vi "Periodic Tasks.vi"(8 "error in":errorcluster) -> ()   [LabVIEW 2013]
doc: "This VI runs in parallel to other tasks. It can contain as many user-defined periodic loops as you need. These can carry out PID or other sorts of timed response."
uses:
  Control 5.ctl
  <vilib>/Rock Robotics/SystemInterfaces/Utilities/FPGA_UtilitiesLED Source.ctl
  <vilib>/Rock Robotics/SystemInterfaces/Utilities/FPGA_UtilitiesLED State.ctl
  Robot Global Data.vi
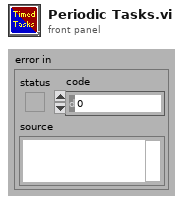
[diagram p1: front panel]
types:
  T1 = typedef "Control 5.ctl" = enum16{"Init", "SetValue", "Disable"}
  T2 = typedef "FPGA_UtilitiesLED State.ctl" = enum16{"Off", "On", "Toggle"}
  T3 = typedef "FPGA_UtilitiesLED Source.ctl" = enum16{"User LED", "FPGA LED"}
  T4 = typedef "WPI_CompressorDevRef.ctl" = cluster{"DevStatus":errorcluster, "DigitalInputDevRef":T5, "RelayDevRef":T8}
  T5 = typedef "WPI_DigitalInputDevRef.ctl" = cluster{"DevStatus":errorcluster, "DIO Channel":T6, "Digital Module":T7}
  T6 = typedef "FPGA_DIOChannel.ctl" = enum8{"DIO 1", "DIO 2", "DIO 3", "DIO 4", "DIO 5", "DIO 6", "DIO 7", "DIO 8", "DIO 9", "DIO 10", "DIO 11", "DIO 12", "DIO 13", "DIO 14", "Invalid"}
  T7 = typedef "FPGA_TypedefDigitalModule.ctl" = enum16{"Digital Module 1", "Digital Module 2"}
  T8 = typedef "WPI_RelayDevRef.ctl" = cluster{"DevStatus":errorcluster, "Relay Channel":T9, "Digital Module":T7, "Relay Direction":T10}
  T9 = typedef "FPGA_DIORelayChannel.ctl" = enum8{"Relay 1", "Relay 2", "Relay 3", "Relay 4", "Relay 5", "Relay 6", "Relay 7", "Relay 8", "Invalid"}
  T10 = typedef "WPI_RelayDirection.ctl" = enum16{"Both directions", "Forward only", "Reverse only"}
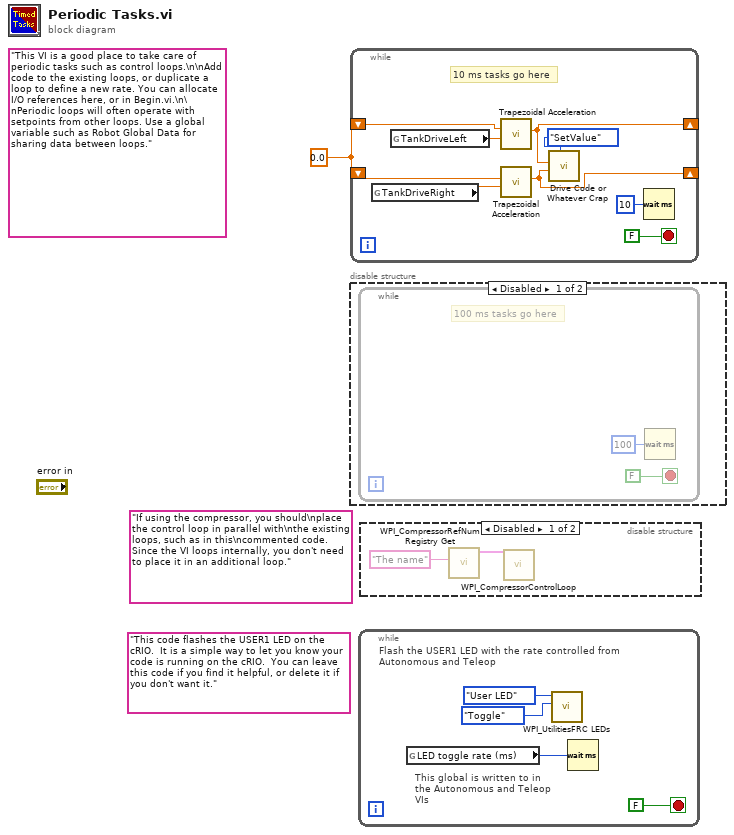
[diagram p0: block diagram]
diagram:
  w1 = 0.0
  (unwired) "If using the compressor, you should\nplace the control loop in parallel with\nthe existing loops, such as in this\ncommented code. Since the VI loops internally, you don't need to place it in an additional loop."
  (unwired) "This code flashes the USER1 LED on the cRIO.  It is a simple way to let you know your code is running on the cRIO.  You can leave this code if you find it helpful, or delete it if you don't want it."
  (unwired) "This VI is a good place to take care of periodic tasks such as control loops.\n\nAdd code to the existing loops, or duplicate a loop to define a new rate. You can allocate I/O references here, or in Begin.vi.\n\nPeriodic loops will often operate with setpoints from other loops. Use a global variable such as Robot Global Data for sharing data between loops."
  n1 = while {
    shift-right: [w3] -> _
    shift-left: w1 -> [w7]
    shift-right: [w2] -> _
    shift-left: w1 -> [w5]
    stop <- FALSE stop-if-true
    # "10 ms tasks go here"
    n2 = global read "Robot Global Data.vi" "TankDriveRight"() -> (w6:dbl)
    n3 = global read "Robot Global Data.vi" "TankDriveLeft"() -> (w8:dbl)
    n4 = call "Trapezoidal Acceleration.vi"("Desired"=w8, "Actual"=w7) -> ("New Actual"=w3:dbl)  [unwired: 9 in]
    n5 = call "Trapezoidal Acceleration.vi"("Desired"=w6, "Actual"=w5) -> ("New Actual"=w2:dbl)  [unwired: 9 in]
    n6 = call "Drive Code or Whatever Crap.vi"("Enum"=Control_5."SetValue", "Right"=w2, "Left"=w3) -> ()  [unwired: 8 in, 1 out]
    n7 = Wait (ms)(milliseconds to wait=u32 10) -> ()  [unwired: 1 out]
  }
  n8 = disable-structure shown="Disabled" {
    frame Disabled {
      n9 = while {
        stop <- FALSE stop-if-true
        # "100 ms tasks go here"
        n10 = Wait (ms)(milliseconds to wait=u32 100) -> ()  [unwired: 1 out]
      }
    }
    frame Enabled {
    }
  }
  n11 = while {
    stop <- FALSE stop-if-true
    # "This global is written to in the Autonomous and Teleop VIs"
    # "Flash the USER1 LED with the rate controlled from Autonomous and Teleop"
    n12 = global read "Robot Global Data.vi" "LED toggle rate (ms)"() -> (w13:u32)
    n13 = call <vilib>:"WPI_UtilitiesFRC LEDs.vi"("State"=FPGA_UtilitiesLED_State."Toggle", "LED Type"=FPGA_UtilitiesLED_Source."User LED") -> ()  [unwired: 1 in, 9 out]
    n14 = Wait (ms)(milliseconds to wait=w13) -> ()  [unwired: 1 out]
  }
  n15 = disable-structure shown="Disabled" {
    frame Disabled {
      n16 = call <vilib>:"WPI_CompressorRefNum Registry Get.vi"("refnum name"="The name") -> ("CompressorDevRef"=w18:T4)  [unwired: 9 in, 1 out]
      n17 = call <vilib>:"WPI_CompressorControlLoop.vi"("CompressorDevRef"=w18) -> ()  [unwired: 11 in]
    }
    frame Enabled {
    }
  }
